vi "SetUnorderedList.vi"(8 "error in (no error)":errorcluster, 10 "OrderedList":refnum<class "Collection.lvclass">, 11 "OrderedList in":refnum<class "UnorderedList.lvclass">) -> (0 "error out":errorcluster, 3 "OrderedList out":refnum<class "UnorderedList.lvclass">)   [LabVIEW 2021, in "Markdown.lvlib" / "UnorderedList.lvclass"]
uses:
  UnorderedList.lvclass
  Collection/Collection.lvclass
  UnorderedList.lvclass/UnorderedList.ctl
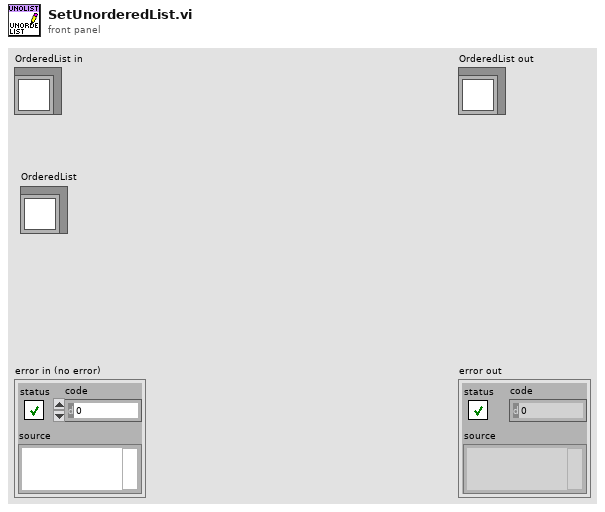
[diagram p1: front panel]
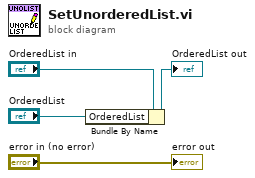
[diagram p0: block diagram]
diagram:
  n1 = Bundle By Name(cluster="OrderedList in", "OrderedList"="OrderedList") -> (→"OrderedList out":refnum<class "UnorderedList.lvclass">)
  "error out" <- "error in (no error)"
